vi "SaveandCloseImage.vi"(8 "error in":errorcluster, 10 "Session In":T1, 11 "Image In":T2(plugin-control)) -> (0 "error out":errorcluster)   [LabVIEW 2017]
uses:
  <vilib>/userdefined/High Color/IMAQdx.ctl
  <vilib>/vision/driver/NI_Vision_Acquisition_Software.lvlib
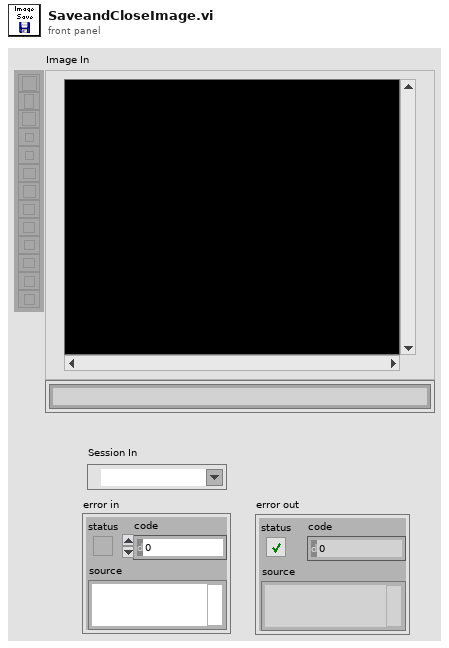
[diagram p1: front panel]
types:
  T1 = typedef "IMAQdx.ctl" = refnum<k21>
  T2 = typedef "IMAQ Image.ctl" = refnum<image>
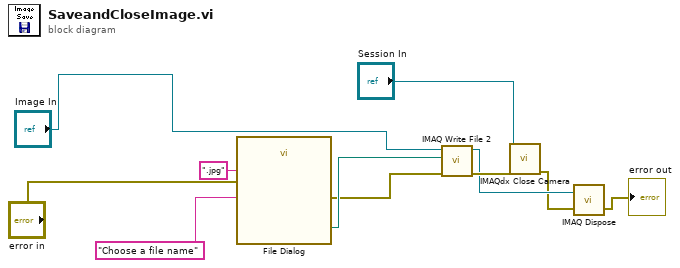
[diagram p0: block diagram]
diagram:
  n1 = call "File Dialog"("prompt"="Choose a file name", "error in"="error in", "pattern (all files)"=".jpg") -> ("selected path"=w8:path, "error out"=w6:errorcluster)  [unwired: 9 in, 2 out]
  n2 = call-poly "IMAQ Write File 2"("error in (no error)"=w6, "File Path"=w8, "Image"="Image In") -> ("error out"=w5:errorcluster, "Image Out (duplicate)"=w3:T2)  [unwired: 7 in]
  n3 = call <vilib>:"IMAQdx Close Camera.vi"("error in"=w5, "Session In"="Session In") -> ("error out"=w2:errorcluster)  [unwired: 9 in]
  n4 = call "IMAQ Dispose"("Image"=w3, "error in (no error)"=w2) -> ("error out"=→"error out":errorcluster)  [unwired: 4 in]
